vi "BonOMM-SAOMM.vi"() -> ()   [LabVIEW 2019] (continued)
                        n3249 = control-ref of="TERMINAL"() -> (w7474:refnum<vi>)
                        n3250 = control-ref of="Indicateur d'état"() -> (w7473:refnum<vi>)
                        n3251 = Concatenate Strings("Chargement de la librairie \"", w7468, "\"") -> (w7471:string)
                        n3252 = call "TERMINAL.vi"("Indicateur Refnum"=w7473, "Terminal Refnum"=w7474, "Indicateur d'état"=w7471) -> ()
                      }
                    }
                  }
                }
              }
              event "modify-librairy": Value Change {
                n3253 = event-data() -> ()  [unwired: 1 in, 6 out]
                n3254 = case shown="Vrai" "modify-librairy" {
                  frame False {
                  }
                  frame True {
                    n3255 = local read "loaded_lib"() -> (w7495:path)
                    n3256 = call "Liste-maker.vi"("Path"=w7495) -> ("Save Path"=w7488:path)
                    n3257 = local read "LST"() -> (w7496:dbl)
                    n3258 = call "Read_obs_files.vi"("Path"=w7488) -> ("path used"=w7487:path, "Output Table"=w7498:string[][])
                    n3259 = for {
                      tunnel: w7498 -> [w7504] mode=indexing
                      tunnel: w7496 -> [w7505]
                      tunnel: [w7501] -> w7497 mode=indexing
                      n3260 = Index Array(array=w7504, index #1=2 ("index"), index #2=3 ("index")) -> (element #1=w7507:string, element #2=w7506:string)
                      n3261 = call "Airmass.vi"("temps sidéral"=w7505, "DEC"=w7506, "RA"=w7507) -> ("airmass"=w7502:dbl)
                      n3262 = Number To Fractional String(number=w7502, precision (6)=i16 2) -> (F-format string=w7503:string)  [unwired: 2 in]
                      n3263 = Insert Into Array(array=w7504, index=5, new element=w7503) -> (w7501:string[])
                    }
                    n3264 = local write "loaded_lib"(w7487) -> ()
                    n3265 = Path To String(path=w7487) -> (string=w7489:string)
                    n3266 = local write "Librairie des objets"(w7497) -> ()
                    n3267 = control-ref of="TERMINAL"() -> (w7491:refnum<vi>)
                    n3268 = control-ref of="Indicateur d'état"() -> (w7490:refnum<vi>)
                    n3269 = Concatenate Strings("Modification de la librairie \"", w7489, "\"") -> (w7494:string)
                    n3270 = call "TERMINAL.vi"("Indicateur Refnum"=w7490, "Terminal Refnum"=w7491, "Indicateur d'état"=w7494) -> ()
                  }
                }
              }
              event "Rechercher...": Mouse Down {
                n3271 = event-data() -> ()  [unwired: 1 in, 8 out]
                n3272 = while {
                  stop <- w7516 continue-if-true
                  n3273 = local read "Librairie complète"() -> (w7511:string[][])
                  n3274 = local read "Rechercher..."() -> (w7514:string)
                  n3275 = call "Update_library.vi"("Librairie des objets"=w7511, "String to Search"=w7514) -> ("lib_out"=w7513:string[][])
                  n3276 = local read "Classé par ..."() -> (w7515:i32)
                  n3277 = Wait (ms)(milliseconds to wait=u32 25) -> ()  [unwired: 1 out]
                  n3278 = call "Sort_table.vi"("Column"=w7515, "Table-In"=w7513) -> ("Table-Out"=w7512:string[][])
                  n3279 = local write "Librairie des objets"(w7512) -> ()
                  n3280 = property on="Rechercher..." class="Ch"() -> ("Key Focus"=w7516:bool)  [unwired: 2 in, 2 out]
                }
              }
              event "Classé par ...": Value Change {
                n3281 = event-data() -> ()  [unwired: 1 in, 6 out]
                n3282 = local read "Librairie des objets"() -> (w7519:string[][])
                n3283 = local read "Classé par ..."() -> (w7517:i32)
                n3284 = call "Sort_table.vi"("Column"=w7517, "Table-In"=w7519) -> ("Table-Out"=w7518:string[][])
                n3285 = local write "Librairie des objets"(w7518) -> ()
              }
              event "centrer_curseur_table": Value Change {
                n3286 = event-data() -> ()  [unwired: 1 in, 6 out]
                n3287 = case shown="Vrai" "centrer_curseur_table" {
                  frame False {
                  }
                  frame True {
                    n3288 = property on="TableXYPos" class="GraphXY (strict)"("Active Cursor"=u32 1 ("Cursor.Cursor Index")) -> (error out=w7524:errorcluster, "Cursor.Cursor Position"=w7522:T45)  [unwired: 2 in, 1 out]
                    n3289 = local write "centrer_curseur_table"(FALSE) -> ()
                    n3290 = property on="TableXYPos" class="GraphXY (strict)"(error in=w7524, "Active Cursor"=u32 0 ("Cursor.Cursor Index"), "Cursor.Cursor Position"=w7522) -> ()  [unwired: 1 in, 2 out]
                  }
                }
              }
              event "centrer_curseur": Value Change {
                n3291 = event-data() -> ()  [unwired: 1 in, 6 out]
                n3292 = local write "centrer_curseur"(FALSE ("centrer_curseur")) -> ()
                n3293 = flat-sequence {
                  frame #0 {
                    n3294 = local write "CursorLock"(TRUE ("CursorLock")) -> ()
                  }
                  frame #1 {
                    n3295 = property on="TableXYPos" class="GraphXY (strict)"() -> ("XScale.Maximum"=w7535:dbl, "XScale.Minimum"=w7534:dbl)  [unwired: 2 in, 2 out]
                    n3296 = property on="TableXYPos" class="GraphXY (strict)"() -> ("YScale.Maximum"=w7531:dbl, "YScale.Minimum"=w7530:dbl)  [unwired: 2 in, 2 out]
                    n3297 = Add(x=w7535, y=w7534) -> (x+y=w7536:dbl)
                    n3298 = Add(x=w7531, y=w7530) -> (x+y=w7532:dbl)
                    n3299 = expression code="x/2"(w7536) -> (w7533:dbl)
                    n3300 = expression code="x/2"(w7532) -> (w7529:dbl)
                    n3301 = property on="TableXYPos" class="GraphXY (strict)"("Active Cursor"=u32 0, "Cursor.Cursor X"=w7533, "Cursor.Cursor Y"=w7529) -> ()  [unwired: 2 in, 2 out]
                  }
                  frame #2 {
                    n3302 = local write "CursorLock"(FALSE ("CursorLock")) -> ()
                  }
                }
              }
              event "SaveExcpt": Value Change {
                n3303 = event-data() -> ()  [unwired: 1 in, 6 out]
                n3304 = case shown="Faux" "SaveExcpt" {
                  frame False {
                  }
                  frame True {
                    n3305 = global read "Globals.vi" "BonOMM VI Refnum"() -> (w7545:refnum<vi>)
                    n3306 = invoke class="VI" method="ValCmde.ToutObt (obs)"(reference=w7545, "controls"=FALSE) -> (reference out=w7544:refnum<vi>, error out=w7543:errorcluster, "Get All Control Values"=w7540:T46)  [unwired: 2 in, 1 out]
                    n3307 = invoke class="VI" method="ValCmde.ToutObt (obs)"(reference=w7544, error in=w7543, "controls"=TRUE) -> ("Get All Control Values"=w7539:T46)  [unwired: 1 in, 3 out]
                    n3308 = call "Save_Params.vi"("Indicators"=w7540, "Controls"=w7539) -> ()  [unwired: 1 in, 1 out]
                  }
                }
              }
              event "Offset RA", "Offset DEC": Value Change; "OffRA_dir", "OffDEC_dir": Mouse Down {
                n3309 = event-data() -> ("CtlRef"=w7553:refnum<vi>)  [unwired: 1 in, 3 out]
                n3310 = property class="Cmde"(reference=w7553) -> ("Label.Text"=w7552:string)  [unwired: 1 in, 2 out]
                n3311 = local read "Offset DEC"() -> (w7550:dbl)
                n3312 = local read "Offset RA"() -> (w7551:dbl)
                n3313 = case shown="\"OffDEC_dir\"" w7552 {
                  tunnel: w7551 -> [w7555 w7556 w7560]
                  tunnel: w7550 -> [w7554 w7558 w7561]
                  tunnel: [w7555 w7556 w7559] -> w7547
                  tunnel: [w7554 w7557 w7561] -> w7546
                  frame "Offset A.D.", "Offset Déc.", Default {
                  }
                  frame "OffDEC_dir" {
                    n3314 = Negate(x=w7558) -> (-x=w7557:dbl)
                    n3315 = local write "Offset DEC"(w7557) -> ()
                    n3316 = local write "Offset RA"(w7556) -> ()
                  }
                  frame "OffRA_dir" {
                    n3317 = Negate(x=w7560) -> (-x=w7559:dbl)
                    n3318 = local write "Offset DEC"(w7561) -> ()
                    n3319 = local write "Offset RA"(w7559) -> ()
                  }
                }
                n3320 = call "Set_Offset_dir.vi"("DEC"=w7546, "RA"=w7547) -> ("DEC_dir"=→"OffDEC_dir":string, "RA_dir"=→"OffRA_dir":string)
              }
              event "Offset RA", "Offset DEC": Mouse Down {
                n3321 = event-data() -> ()  [unwired: 1 in, 8 out]
              }
              event "copy_calib", "copy_ref", "copy_centre": Value Change {
                n3322 = event-data() -> ("CtlRef"=w7570:refnum<vi>)  [unwired: 1 in, 5 out]
                n3323 = property class="Bool"(reference=w7570) -> ("Label.Text"=w7569:string)  [unwired: 1 in, 2 out]
                n3324 = case shown="\"copy_ref\"" w7569 {
                  tunnel: ["<NO REFERENCE>" "de calibration" "de la référence instrumentale" "du centre optique"] -> w7565
                  frame Default {
                  }
                  frame "copy_calib" {
                  }
                  frame "copy_ref" {
                  }
                  frame "copy_centre" {
                  }
                }
                n3325 = Concatenate Strings("Êtes vous certain de vouloir modifier la position ", w7565, " ?") -> (w7564:string)
                n3326 = Two Button Dialog(message=w7564, 1:"NON" ("T button name (\"OK\")"), 2:"OUI" ("T button name (\"OK\")")) -> (T button?=w7568:bool)
                n3327 = case shown="Vrai" w7568 {
                  tunnel: w7569 -> [_ w7571]
                  frame False {
                  }
                  frame True {
                    n3328 = local read "Position X"() -> (w7574:dbl)
                    n3329 = local read "Position Y"() -> (w7573:dbl)
                    n3330 = local read "Position Z"() -> (w7572:dbl)
                    n3331 = case shown="\"copy_centre\"" w7571 {
                      tunnel: w7574 -> [_ w7576 w7578 w7580]
                      tunnel: w7573 -> [_ w7575 w7577 w7579]
                      tunnel: w7572 -> [_ _ _ _]
                      frame Default {
                      }
                      frame "copy_calib" {
                        n3332 = local write "Calibration X"(w7576) -> ()
                        n3333 = local write "Calibration Y"(w7575) -> ()
                      }
                      frame "copy_ref" {
                        n3334 = local write "Reference X"(w7578) -> ()
                        n3335 = local write "Reference Y"(w7577) -> ()
                      }
                      frame "copy_centre" {
                        n3336 = local write "CentreTel X"(w7580) -> ()
                        n3337 = local write "CentreTel Y"(w7579) -> ()
                      }
                    }
                  }
                }
              }
              event "Cen-Snd-RA", "Cen-Snd-DEC", "Cen-Cib-RA", "Cen-Cib-DEC": Value Change {
                n3338 = event-data() -> ()  [unwired: 1 in, 6 out]
                n3339 = disable-structure shown="Disabled" {
                  frame Disabled {
                    n3340 = local read "Cen-Snd-DEC"() -> ()  [unwired: 1 out]
                    n3341 = local read "Cen-Snd-RA"() -> ()  [unwired: 1 out]
                  }
                  frame Enabled {
                  }
                }
                n3342 = call "format_string2arcmin.vi"("Arcmin-Str"="Cen-Cib-DEC") -> ("Arcmin"=w7588:dbl)  [unwired: 14 in]
                n3343 = call "format_string2arcmin.vi"("Arcmin-Str"="Cen-Cib-RA") -> ("Arcmin"=w7589:dbl)  [unwired: 14 in]
                n3344 = property on="TableXYPos" class="GraphXY (strict)"("Active Cursor"=u32 0, "Cursor.Cursor X"=w7589, "Cursor.Cursor Y"=w7588) -> ()  [unwired: 2 in, 2 out]
              }
              event "best_target": Value Change {
                # "Remettre les conditions sur BestTargetLed"
                n3345 = event-data() -> ()  [unwired: 1 in, 6 out]
                n3346 = stacked-sequence {
                  frame #0 {
                    n3347 = local write "best_target"(FALSE ("best_target")) -> ()
                    n3348 = property on="best_target" class="Bool (strict)"("DisabledEnum"=T17."Disabled" ("Disabled")) -> ()  [unwired: 2 in, 2 out]
                  }
                  frame #1 {
                    # "Vérifie si le data est à date ..."
                    n3349 = local read "BestTargetLed"() -> (w7592:bool)
                    n3350 = case shown="Faux" w7592 {
                      frame False {
                        n3351 = local read "DEC-Champ"() -> (w7594:dbl)
                        n3352 = local read "RA-Champ"() -> (w7595:dbl)
                        n3353 = local write "BestTargetLed"(FALSE ("BestTargetLed")) -> ()
                        n3354 = flat-sequence {
                          tunnel: [w7604] -> w7596
                          tunnel: w7595 -> [w7601]
                          tunnel: w7594 -> [w7600]
                          tunnel: w7596 -> [w7622]
                          frame #0 {
                            # "R1mag limite USNO"
                            n3355 = local read "Représentation"() -> (w7599:dbl)
                            n3356 = local read "path_data"() -> (w7606:path)
                            n3357 = local read "wgetexec"() -> (w7605:path)
                            n3358 = Add(x=w7599, y=10.0) -> (x+y=w7597:dbl)
                            n3359 = while {
                              stop <- w7610 stop-if-true
                              n3360 = local read "BestTargetLed"() -> (w7612:bool)
                              n3361 = Wait (ms)(milliseconds to wait=u32 333) -> ()  [unwired: 1 out]
                              n3362 = Not(x=w7612) -> (.not. x?=w7611:bool)
                              n3363 = local write "BestTargetLed"(w7611) -> ()
                              n3364 = local read "USNO_ready"() -> (w7610:bool)
                            }
                            n3365 = call "QueryUSNO.vi"("wget"=w7605, "Data dir Path"=w7606, "mag_limit"=12.0, "radius"=w7597, "DEC"=w7600, "RA"=w7601) -> ("Data OUT"=w7607:string[][], "No Error"=w7602:bool)  [unwired: 3 in, 1 out]
                            n3366 = case shown="Vrai" w7602 {
                              tunnel: w7607 -> [_ w7621]
                              tunnel: w7602 -> [w7614 w7619]
                              tunnel: [w7614 w7619] -> w7604
                              tunnel: [TRUE TRUE] -> w7603
                              tunnel: w7601 -> [_ w7616]
                              tunnel: w7600 -> [_ w7615]
                              frame False {
                              }
                              frame True {
                                # "6 = R1mag"
                                n3367 = call "Sort_USNO_data.vi"("Column Used"=6, "Data IN"=w7621) -> ("Data OUT"=w7617:string[][])  [unwired: 8 in, 1 out]
                                n3368 = local write "USNO_data"(w7617) -> ()
                                "RA-USNO" <- w7616
                                "DEC-USNO" <- w7615
                              }
                            }
                            n3369 = local write "USNO_ready"(w7603) -> ()
                          }
                          frame #1 {
                            n3370 = local write "USNO_ready"(w7622) -> ()
                            "BestTargetLed" <- w7622
                          }
                        }
                      }
                      frame True {
                      }
                    }
                  }
                  frame #2 {
                    n3371 = local read "BestTargetLed"() -> (w7623:bool)
                    n3372 = case shown="Vrai" w7623 {
                      frame False {
                      }
                      frame True {
                        w7624 = u16 1 items=["Region d'intérêt", "Prévisualisation", "Idle"] ("ImageUsage")
                        # "Proper motion limit (mas/yr)"
                        # "Pickup mirror footprint (arcmin)"
                        # "R1mag lower limit"
                        n3373 = local read "FOV"() -> (w7652:dbl)
                        n3374 = local read "TableAstrom"() -> (w7635:T4)
                        n3375 = local read "USNO_data"() -> (w7657:string[][])
                        n3376 = local read "Epoch Tel"() -> (w7654:dbl)
                        n3377 = local read "DEC Tel"() -> (w7655:dbl)
                        n3378 = local read "RA Tel"() -> (w7656:dbl)
                        n3379 = call "Choose_best_target(multi).vi"("R1mag lower limit"=6.0, "FOV"=w7652, "Footprint"=1.0, "PM limit"=25.0 ("Footprint"), "EPOCH TEL"=w7654, "DEC TEL"=w7655, "Table Astrometry"=w7635, "RA TEL"=w7656, "USNO_data"=w7657) -> ("Best Target"=w7634:string[][], "target RA (deg)"=w7643:dbl, "target DEC (deg)"=w7642:dbl)  [unwired: 3 in, 5 out]
                        "Target Data" <- w7634
                        n3380 = local read "FirstBest"() -> (w7641:bool)
                        n3381 = case shown="Faux" w7641 {
                          selector: w7641 -> [_ w7675]
                          tunnel: w7643 -> [_ w7677]
                          tunnel: [w7661 w7677] -> w7631
                          tunnel: w7642 -> [_ w7676]
                          tunnel: [w7660 w7676] -> w7630
                          tunnel: w7634 -> [w7672 _]
                          frame False {
                            n3382 = Increment(x="BestCount") -> (x+1=w7668:i32)
                            n3383 = Index Array(array=w7672, index (row)="BestCount") -> (element=w7669:string[])  [unwired: 1 in]
                            n3384 = Quotient & Remainder(x=w7668, y=3) -> (x-y*floor(x/y)=w7671:i32)  [unwired: 1 out]
                            n3385 = Index Array(array=w7669) -> (element #1=w7667:string, element #2=w7666:string, element #3=w7665:string)  [unwired: 3 in]
                            n3386 = local read "Epoch Tel"() -> (w7658:dbl)
                            n3387 = Fract/Exp String To Number(string=w7667) -> (number=w7664:dbl)  [unwired: 3 in, 1 out]
                            n3388 = Fract/Exp String To Number(string=w7666) -> (number=w7663:dbl)  [unwired: 3 in, 1 out]
                            n3389 = Fract/Exp String To Number(string=w7665) -> (number=w7662:dbl)  [unwired: 3 in, 1 out]
                            n3390 = local write "BestCount"(w7671) -> ()
                            n3391 = call "precess.vi"("Eq2"=w7658, "Eq1"=w7662, "DEC 1"=w7663, "RA 1"=w7664) -> ("DEC 2"=w7660:dbl, "RA 2"=w7661:dbl)
                          }
                          frame True {
                            n3392 = Not(x=w7675) -> (.not. x?=→"FirstBest":bool)
                            n3393 = local write "BestCount"(1 ("BestCount")) -> ()
                          }
                        }
                        n3394 = local read "ImageDSSLed"() -> (w7644:bool)
                        n3395 = local read "Epoch Tel"() -> (w7628:dbl)
                        n3396 = call "precess.vi"("Eq2"=2000.0, "Eq1"=w7628, "DEC 1"=w7630, "RA 1"=w7631) -> ("DEC 2"=w7626:dbl, "RA 2"=w7627:dbl)
                        n3397 = call "deg2ad.vi"("DEC (°)"=w7630, "RA (°)"=w7631) -> ("DEC (°)"=→"RA-USNO-sec 3":dbl, "RA (sec)"=→"RA-USNO-sec 2":dbl)
                        n3398 = case shown="Faux" w7644 {
                          tunnel: w7627 -> [w7682 w7701]
                          tunnel: w7626 -> [w7681 w7700]
                          tunnel: [w7679 w7699] -> w7646
                          frame False {
                            w7683 = 2.0 ("Size")
                            n3399 = local read "wgetexec"() -> (w7685:path)
                            n3400 = local read "path_dss"() -> (w7684:path)
                            n3401 = call "Query_Vizier.vi"("Folder"=w7684, "wget"=w7685, "Width"=w7683, "Height"=w7683, "DEC"=w7681, "RA"=w7682) -> ("error?"=w7678:bool, "Path2Image"=w7680:path)  [unwired: 4 in]
                            n3402 = case shown="Faux" w7678 {
                              tunnel: w7680 -> [w7690 _]
                              tunnel: [w7689 w7697] -> w7679
                              frame False {
                                n3403 = call "gfitsio-open-create-replace-file.vi"("file path (dialog if empty)"=w7690) -> ("error out"=w7695:errorcluster, "gfits refnum"=w7694:T47)  [unwired: 8 in, 1 out]
                                n3404 = call "gfitsio-read-header.vi"("error in (no error)"=w7695, "gfits refnum"=w7694) -> ("error out"=w7692:errorcluster, "dup gfits refnum"=w7693:T47)  [unwired: 7 in, 1 out]
                                n3405 = call-poly "gfitsio-read-image-subset.vi"("lpixel (-1,-1: rest)"=cluster{"X":i32, "Y":i32} {"X"=-1, "Y"=-1}, "fpixel (1,1)"=cluster{"X":i32, "Y":i32} {"X"=1, "Y"=1}, "error in (no error)"=w7692, "gfits refnum"=w7693) -> ("error out"=w7688:errorcluster, "data"=w7689:sgl[][], "dup gfits refnum"=w7687:T47)  [unwired: 4 in, 1 out]
                                n3406 = call "gfitsio-close-file.vi"("error in (no error)"=w7688, "gfits refnum"=w7687) -> ("error out"=→"fits Error":errorcluster)  [unwired: 8 in, 1 out]
                              }
                              frame True {
                                w7698 = sgl 0.0 ("element")
                                n3407 = Initialize Array(w7698, w7698, w7698) -> (w7697:sgl[][])
                              }
                            }
                          }
                          frame True {
                            n3408 = local read "ImgAstrom"() -> (w7709:T4)
                            n3409 = call "ad2xy.vi"("DEC"=w7700, "RA"=w7701, "Astrometry"=w7709) -> ("Y"=w7706:dbl, "X"=w7707:dbl)  [unwired: 6 in, 1 out]
                            n3410 = To Long Integer(number=w7707) -> (32bit integer=w7705:i32)
                            n3411 = To Long Integer(number=w7706) -> (32bit integer=w7704:i32)
                            n3412 = local read "ImgData"() -> (w7708:sgl[][])
                            n3413 = call "subimage.vi"("Ysz/2"=100, "Xsz/2"=100, "Yc"=w7704, "Xc"=w7705, "ImgData"=w7708) -> ("SubImg"=w7699:sgl[][])  [unwired: 6 in]
                          }
                        }
                        n3414 = local read "FieldAstrom"() -> (w7648:T4)
                        n3415 = local write "SubIMG4DSS?"(TRUE ("SubIMG4DSS?")) -> ()
                        n3416 = call "ad2xy.vi"("DEC"=w7630, "RA"=w7631, "Astrometry"=w7648) -> ("Y"=w7636:dbl, "X"=w7637:dbl)  [unwired: 6 in, 1 out]
                        n3417 = property on="TableXYPos" class="GraphXY (strict)"("Active Cursor"=u32 0, "Cursor.Cursor Position:Cursor X"=w7637, "Cursor.Cursor Position:Cursor Y"=w7636) -> ()  [unwired: 2 in, 2 out]
                        n3418 = call "format_arcmin2arcsecstr.vi"("RA arcmin"=w7637, "DEC Arcmin"=w7636) -> ("Formatted RA"=w7640:string, "Formatted Dist"=w7638:string, "Formatted DEC"=w7639:string)  [unwired: 11 in]
                        n3419 = Array Max & Min(array=w7646) -> (max value=w7647:sgl)  [unwired: 3 out]
                        n3420 = call "Draw_crosshair.vi"("Image IN"=w7646, "White Value"=w7647) -> ("Image OUT"=w7645:sgl[][])  [unwired: 13 in]
                        n3421 = local write "Cen-Cib-TOT"(w7638) -> ()
                        n3422 = local write "Cen-Cib-RA"(w7640) -> ()
                        n3423 = local write "Cen-Cib-DEC"(w7639) -> ()
                        n3424 = local write "ImageUsage"(w7624) -> ()
                        n3425 = local write "subimg"(w7645) -> ()
                      }
                    }
                  }
                  frame #3 {
                    n3426 = property on="best_target" class="Bool (strict)"("DisabledEnum"=T17."Enabled" ("Disabled")) -> ()  [unwired: 2 in, 2 out]
                  }
                }
              }
              event "GetDSS", "DS9": Value Change {
                # "Trace l'image DSS par dessus le champ des tables de guidage"
                n3427 = event-data() -> ("CtlRef"=w7715:refnum<vi>)  [unwired: 1 in, 4 out]
                n3428 = flat-sequence {
                  tunnel: w7715 -> [w7721]
                  tunnel: [w7720] -> w7714
                  tunnel: [w7753] -> w7717
                  tunnel: w7714 -> [w7747]
                  tunnel: [w7741] -> w7713
                  tunnel: [w7740] -> w7712
                  tunnel: [w7739] -> w7711
                  tunnel: w7717 -> [w7810]
                  tunnel: path "C:/BonOMM/BonOMM-2012/Apps/SAOImage-DS9/ds9.exe" ("DS9path") -> [w7809]
                  tunnel: w7713 -> [w7805]
                  tunnel: w7712 -> [w7807]
                  tunnel: w7711 -> [w7806]
                  frame #0 {
                    w7719 = T17."Disabled" ("Disabled")
                    w7718 = FALSE ("DSS_ready")
                    n3429 = property class="Bool (strict)"(reference=w7721) -> ("Label.Text"=w7720:string)  [unwired: 1 in, 2 out]
                    n3430 = local write "ImageDSSLed"(w7718) -> ()
                    n3431 = local write "DS9-Led"(w7718) -> ()
                    n3432 = local write "DSS_ready"(w7718) -> ()
                    n3433 = local write "DS9_ready"(w7718) -> ()
                    n3434 = local write "GetDSS"(w7718) -> ()
                    n3435 = property on="DS9" class="Bool (strict)"("DisabledEnum"=w7719) -> ()  [unwired: 2 in, 2 out]
                    n3436 = property on="GetDSS" class="Bool (strict)"("DisabledEnum"=w7719) -> ()  [unwired: 2 in, 2 out]
                    n3437 = local write "DS9"(w7718) -> ()
                  }
                  frame #1 {
                    w7772 = u16 0 items=["Square", "Circle"] ("Ring")
                    # "Invert X"
                    # "Époque DSS et USNO"
                    n3438 = local read "Reference Y"() -> (w7774:dbl)
                    n3439 = local read "Reference X"() -> (w7773:dbl)
                    n3440 = local read "CentreTel X"() -> (w7737:dbl)
                    n3441 = local read "CentreTel Y"() -> (w7736:dbl)
                    n3442 = local read "RotationEffective"() -> (w7733:dbl)
                    n3443 = local read "arcsec/pulse"() -> (w7770:dbl)
                    n3444 = local read "Représentation"() -> (w7746:dbl)
                    n3445 = To Double Precision Float(number=w7773) -> (double precision float=w7765:dbl)
                    n3446 = To Double Precision Float(number=w7774) -> (double precision float=w7764:dbl)
                    n3447 = Equal?(x=w7747, y="DS9") -> (x = y?=w7741:bool)
                    n3448 = Select(t=60.0, s=w7741, f=w7746) -> (s? t:f=w7745:dbl)
                    n3449 = local read "DEC Tel"() -> (w7767:dbl)
                    n3450 = local read "RA Tel"() -> (w7766:dbl)
                    n3451 = while {
                      tunnel: w7747 -> [w7775]
                      stop <- w7777 stop-if-true
                      n3452 = case shown="\"DS9\"" w7775 {
                        tunnel: [TRUE ("DSS_ready") w7781 "DS9_ready"] -> w7777
                        frame "False", Default {
                        }
                        frame "GetDSS" {
                          n3453 = local read "ImageDSSLed"() -> (w7779:bool)
                          n3454 = local read "DSS_ready"() -> (w7781:bool)
                          n3455 = Not(x=w7779) -> (.not. x?=→"ImageDSSLed":bool)
                        }
                        frame "DS9" {
                          n3456 = local read "DS9-Led"() -> (w7783:bool)
                          n3457 = Not(x=w7783) -> (.not. x?=→"DS9-Led":bool)
                        }
                      }
                      n3458 = Wait (ms)(milliseconds to wait=u32 333) -> ()  [unwired: 1 out]
                    }
                    n3459 = call "Set_field_astrometry.vi"("Cen x (pas)"=w7737, "effective rotation (°)"=w7733, "scale (\"/pas)"=w7770, "NaxisMax"=500000, "Cen y (pas)"=w7736, "Use Center?"=FALSE ("Ues Constant Size ?"), "Ref x (pas)"=w7765, "Ref y (pas)"=w7764, "RA (HH:MM:SS.S)"=w7766, "DEC(DD:MM:SS)"=w7767, "Inversion Cluster"=T20 {"Invert Angle"=FALSE, "Invert X"=TRUE, "Invert Y"=FALSE}) -> ("Field Astrometry"=w7759:T4, "Table Astrometry"=w7760:T4)  [unwired: 3 in]
                    n3460 = local read "MirVig"() -> (w7730:dbl)
                    n3461 = property on="TableXYPos" class="GraphXY (strict)"("Active Cursor"=u32 1) -> ("Cursor.Cursor X"=w7728:dbl, "Cursor.Cursor Y"=w7729:dbl)  [unwired: 2 in, 2 out]
                    n3462 = local read "BrasPesto"() -> (w7722:bool)
                    n3463 = local read "LimXPesto"() -> (w7723:dbl)
                    n3464 = local read "MirFOV"() -> (w7725:dbl)
                    n3465 = local read "Miroir"() -> (w7727:dbl)
                    n3466 = local read "FOV"() -> (w7771:dbl)
                    n3467 = local write "TableAstrom"(w7760) -> ()
                    n3468 = local read "NaxisMax"() -> (w7738:dbl)
                    n3469 = Bundle("Miroir"=w7727, "Cursor.Cursor X"=w7728, "Cursor.Cursor Y"=w7729, "MirVig"=w7730, "MirFOV"=w7725, "LimXPesto"=w7723, "BrasPesto"=w7722) -> (w7726:T48)  [unwired: 1 in]
                    n3470 = local read "RotationEffective"() -> (w7724:dbl)
                    n3471 = local read "Epoch Tel"() -> (w7757:dbl)
                    n3472 = call "draw_field.vi"("Field_Astrometry"=w7759, "FOV"=w7771, "NaxisMax"=w7738, "Ring"=w7772, "Table_Astrometry"=w7760, "Rotation effective"=w7724, "Ues Constant Size ?"=TRUE, "margin/size"=w7745, "MirrorAvatar"=w7726) -> ("X Scale.Range"=w7752:T26, "ImgDEC"=w7732:dbl, "ImgRA"=w7756:dbl, "Y Scale.Range"=w7751:T26)  [unwired: 2 in, 1 out]
                    n3473 = call "precess.vi"("Eq2"=2000.0, "Eq1"=w7757, "DEC 1"=w7732, "RA 1"=w7756) -> ("DEC 2"=w7754:dbl, "RA 2"=w7755:dbl)
                    n3474 = local read "path_dss"() -> (w7762:path)
                    n3475 = Add(x=w7745, y=4.0) -> (x+y=w7750:dbl)
                    n3476 = local read "wgetexec"() -> (w7761:path)
                    n3477 = local write "FieldAstrom"(w7759) -> ()
                    n3478 = call "Query_Vizier.vi"("Folder"=w7762, "wget"=w7761, "Width"=w7750, "Height"=w7750, "DEC"=w7754, "RA"=w7755) -> ("error?"=w7742:bool, "Path2Image"=w7763:path)  [unwired: 4 in]
                    n3479 = local write "Img DEC"(w7754) -> ()
                    n3480 = local write "Img RA"(w7755) -> ()
                    n3481 = Or(x=w7742, y=w7741) -> (x .or. y?=w7743:bool)
                    n3482 = case shown="Faux" w7743 {
                      tunnel: w7755 -> [w7797 _]
                      tunnel: w7754 -> [w7796 _]
                      tunnel: w7763 -> [w7788 w7803]
                      tunnel: w7759 -> [w7794 _]
                      tunnel: [TRUE TRUE] -> w7740
                      tunnel: [w7788 w7803] -> w7753
                      tunnel: w7752 -> [w7787 _]
                      tunnel: w7751 -> [w7786 _]
                      tunnel: [w7785 FALSE] -> w7739
                      frame False {
                        # "ImgData et ImgAstrom\nsont lié à plus grand que le\nchamp affiché."
                        n3483 = property on="TableXYPos" class="GraphXY (strict)"() -> ("Height"=w7801:u32, "Width"=w7800:u32)  [unwired: 2 in, 2 out]
                        n3484 = To Long Integer(number=w7801) -> (32bit integer=w7799:i32)
                        n3485 = To Long Integer(number=w7800) -> (32bit integer=w7798:i32)
                        n3486 = call "Draw_graph_background.vi"("Y Scale.Range"=w7786, "ImgRA"=w7797, "X Scale.Range"=w7787, "ImgDEC"=w7796, "Field Astrometry"=w7794, "New Width"=w7798, "New Height"=w7799, "path"=w7788) -> ("ImgData"=w7789:sgl[][], "Astrometry"=w7793:T4, "error out"=w7791:errorcluster, "Images"=w7795:picture)
                        "DSS Error" <- w7791
                        n3487 = Unbundle By Name(w7791) -> ("status"=w7790:bool)
                        n3488 = property on="TableXYPos" class="GraphXY (strict)"("PlotImages.Back"=w7795) -> ()  [unwired: 2 in, 2 out]
                        n3489 = local write "ImgAstrom"(w7793) -> ()
                        n3490 = local write "ImgData"(w7789) -> ()
                        n3491 = Not(x=w7790) -> (.not. x?=w7785:bool)
                      }
                      frame True {
                      }
                    }
                    n3492 = local write "DSS_ready"(w7740) -> ()
                    n3493 = local write "DS9_ready"(w7740) -> ()
                  }
                  frame #2 {
                    w7808 = T17."Enabled" ("Disabled")
                    n3494 = property on="GetDSS" class="Bool (strict)"("DisabledEnum"=w7808) -> ()  [unwired: 2 in, 2 out]
                    n3495 = case shown="Vrai" w7805 {
                      tunnel: w7810 -> [_ w7814]
                      tunnel: w7809 -> [_ w7813]
                      tunnel: w7807 -> [_ w7812]
                      tunnel: w7806 -> [w7811 _]
                      frame False {
                        n3496 = local write "ImageDSSLed"(w7811) -> ()
                      }
                      frame True {
                        n3497 = local write "DS9-Led"(w7812) -> ()
                        n3498 = call "fits2ds9.vi"("DS9path"=w7813, "FitsFile"=w7814) -> ()  [unwired: 10 in]
                      }
                    }
                    n3499 = property on="DS9" class="Bool (strict)"("DisabledEnum"=w7808) -> ()  [unwired: 2 in, 2 out]
                  }
                }
              }
              event "BoutonTest": Value Change {
                n3500 = event-data() -> ()  [unwired: 1 in, 6 out]
                n3501 = flat-sequence {
                  frame #0 {
                    n3502 = local write "QueryingHexapod"(TRUE ("QueryingHexapod")) -> ()
                    n3503 = property on="HexapodRefresh" class="Bool (strict)"("Val(Sgnl)"=TRUE ("Valeur (Signalisation)")) -> ()  [unwired: 2 in, 2 out]
                  }
                  frame #1 {
                    n3504 = while {
                      i -> [w7821]
                      stop <- w7818 stop-if-true
                      n3505 = local read "QueryingHexapod"() -> (w7822:bool)
                      n3506 = Not(x=w7822) -> (.not. x?=w7820:bool)
                      n3507 = call "Max-iteration.vi"("i max"=50, "i act"=w7821, "Valeur entrante"=w7820) -> ("break ?"=w7818:bool)
                      n3508 = Wait (ms)(milliseconds to wait=u32 100 ("attente (ms)")) -> ()  [unwired: 1 out]
                    }
                    n3509 = local write "GE_Hex_X"(0.01 ("GE_Hex_X")) -> ()
                  }
                  frame #2 {
                    n3510 = local read "GE_Hex_Y"() -> (w7828:dbl)
                    n3511 = local read "GE_Hex_U"() -> (w7826:dbl)
                    n3512 = local read "GE_Hex_X"() -> (w7829:dbl)
                    n3513 = local read "GE_Hex_Z"() -> (w7827:dbl)
                    n3514 = local read "GE_Hex_V"() -> (w7825:dbl)
                    n3515 = local read "Hexapod VRN"() -> (w7833:refnum<visa-resource-name>)
                    n3516 = control-ref of="HexX"() -> (w7840:refnum<vi>)
                    n3517 = control-ref of="HexY"() -> (w7839:refnum<vi>)
                    n3518 = control-ref of="HexU"() -> (w7837:refnum<vi>)
                    n3519 = control-ref of="HexV"() -> (w7836:refnum<vi>)
                    n3520 = control-ref of="HexZ"() -> (w7838:refnum<vi>)
                    n3521 = control-ref of="Hexapod-ACK"() -> (w7831:refnum<vi>)
                    n3522 = control-ref of="HexaCons actif"() -> (w7832:refnum<vi>)
                    n3523 = local read "MessageType"() -> (w7834:cluster{string[], u32[]})
                    n3524 = Bundle("GE_Hex_X"=w7829, "GE_Hex_Y"=w7828, "GE_Hex_Z"=w7827, "GE_Hex_U"=w7826, "GE_Hex_V"=w7825) -> (w7824:T49)  [unwired: 1 in]
                    n3525 = Bundle("HexX"=w7840, "HexY"=w7839, "HexZ"=w7838, "HexU"=w7837, "HexV"=w7836) -> (w7835:T29)  [unwired: 1 in]
                    n3526 = call "TEST-SAOMM-Externaloffset.vi"("Hexapod VRN"=w7833, "Active Refnum"=w7832, "PrAMS-ACK"=w7831, "output cluster"=w7835, "offset_cluster"=w7824, "MessageType"=w7834) -> ("Error"=w7830:bool)  [unwired: 9 in]
                    n3527 = case shown="Vrai" w7830 {
                      frame False {
                      }
                      frame True {
                        n3528 = One Button Dialog(message="Erreur lors de l'envoi des valeurs offset 2") -> ()  [unwired: 1 in, 1 out]
                      }
                    }
                  }
                }
              }
              event "LVDT-Set-ZERO": Value Change {
                n3529 = event-data() -> ()  [unwired: 1 in, 5 out]
                n3530 = local write "LVDT-Set-ZERO"(FALSE ("LVDT-Set-ZERO")) -> ()
                n3531 = flat-sequence {
                  tunnel: [w7846] -> w7842
                  tunnel: w7842 -> [w7847]
                  frame #0 {
                    n3532 = Two Button Dialog(message="Assurez-vous que les moteurs sont éteints depuis au\nmoins 30 secondes et que les plateaux sont bien engagés.", 1:"Annuler" ("F button name (\"Cancel\")")) -> (T button?=w7846:bool)  [unwired: 1 in]
                  }
                  frame #1 {
                    n3533 = case shown="Vrai" w7847 {
                      frame False {
                      }
                      frame True {
                        n3534 = local read "Graph Data"() -> (w7848:dbl[])
                        n3535 = call-poly <vilib>:"Mean.vi"("X"=w7848) -> ("mean"=w7849:dbl)  [unwired: 1 out]
                        n3536 = local write "LVDT-zero"(w7849) -> ()
                      }
                    }
                  }
                }
              }
              event "LVDT-Save-Data": Value Change {
                n3537 = event-data() -> ()  [unwired: 1 in, 5 out]
                n3538 = local write "LVDT-Save-Data"(FALSE ("want seconds? (F)")) -> ()
                n3539 = local read "LVDT-RA-Data"() -> (w7875:dbl[])
                n3540 = local read "Q String"() -> (w7871:string)
                n3541 = Array To Spreadsheet String(delimiter (Tab)="\n", array=w7875, 3:"%5f") -> (spreadsheet string=w7873:string)
                n3542 = Get Date/Time String(date format (0)=enum16{"short", "long", "abbreviated"}."short", want seconds? (F)=TRUE) -> (date string=w7859:string, time string=w7854:string)  [unwired: 1 in]
                n3543 = local read "path_syslogs"() -> (w7869:path)
                n3544 = Search and Replace String(replace all?=TRUE ("replace all? (F)"), input string=w7859, search string="-") -> (result string=w7853:string)  [unwired: 5 in, 3 out]
                n3545 = Search and Replace String(replace all?=TRUE ("replace all? (F)"), input string=w7854, search string=":") -> (result string=w7852:string)  [unwired: 5 in, 3 out]
                n3546 = Concatenate Strings(w7871, "\n\n***\n\n", w7873) -> (w7870:string)
                n3547 = Concatenate Strings(w7853, w7852, ".lvdt" ("name or relative path")) -> (w7862:string)
                n3548 = Build Path(base path=w7869, name or relative path="LVDTs") -> (appended path=w7867:path)
                n3549 = local read "File I/O Error"() -> (w7861:errorcluster)
                n3550 = Build Path(base path=w7867, name or relative path=w7862) -> (appended path=w7866:path)
                n3551 = Write to Text File(file (use dialog)=w7866, text=w7870, error in=w7861) -> (error out=w7860:errorcluster)  [unwired: 1 in, 2 out]
                n3552 = local write "File I/O Error"(w7860) -> ()
              }
              event "SpliterSelector": Value Change {
                n3553 = event-data() -> ("OldVal"=w7878:u16, "NewVal"=w7877:u16)  [unwired: 1 in, 3 out]
                n3554 = Not Equal?(x=w7878, y=w7877) -> (x != y?=w7876:bool)
                n3555 = case shown="Vrai" w7876 {
                  frame False {
                  }
                  frame True {
                    n3556 = flat-sequence {
                      frame #0 {
                        "SplitterMoving" <- TRUE
                      }
                      frame #1 {
                        n3557 = flat-sequence {
                          tunnel: "SpliterSelector" -> [w7885]
                          frame #0 {
                            n3558 = case shown="1" w7885 {
                              tunnel: [w7886 w7891 w7892] -> _
                              frame 2 {
                                w7888 = u16 1 items=["Initialisation", "Mise dans le faisceau", "Retirer du faisceau"] ("Commande")
                                n3559 = local read "Splitter VRN"() -> (w7887:refnum<visa-resource-name>)
                                n3560 = call "MicroSlide-Execute.vi"("VISA resource name"=w7887, "Commande"=w7888) -> ("Error OUT"=w7886:errorcluster)  [unwired: 10 in, 3 out]
                              }
                              frame 0, Default {
                                w7889 = u16 0 items=["Initialisation", "Mise dans le faisceau", "Retirer du faisceau"] ("Commande")
                                n3561 = local read "Splitter VRN"() -> (w7890:refnum<visa-resource-name>)
                                n3562 = call "MicroSlide-Execute.vi"("VISA resource name"=w7890, "Commande"=w7889) -> ("Error OUT"=w7891:errorcluster)  [unwired: 10 in, 3 out]
                              }
                              frame 1 {
                                w7894 = u16 2 items=["Initialisation", "Mise dans le faisceau", "Retirer du faisceau"] ("Commande")
                                n3563 = local read "Splitter VRN"() -> (w7893:refnum<visa-resource-name>)
                                n3564 = call "MicroSlide-Execute.vi"("VISA resource name"=w7893, "Commande"=w7894) -> ("Error OUT"=w7892:errorcluster)  [unwired: 10 in, 3 out]
                              }
                            }
                          }
                          frame #1 {
                            n3565 = local write "SplitterMoving"(FALSE ("SplitterMoving")) -> ()
                          }
                        }
                        n3566 = while {
                          stop <- w7884 continue-if-true
                          n3567 = local read "SpliterIndic"() -> (w7881:bool)
                          n3568 = Wait (ms)(milliseconds to wait=u32 250) -> ()  [unwired: 1 out]
                          n3569 = Not(x=w7881) -> (.not. x?=→"SpliterIndic":bool)
                          n3570 = local read "SplitterMoving"() -> (w7884:bool)
                        }
                      }
                      frame #2 {
                        # "À mettre en gestion d'erreur"
                        n3571 = local write "SpliterIndic"(TRUE ("SpliterIndic")) -> ()
                      }
                    }
                  }
                }
              }
            }
          }
          "Événements Usagés" <- w982
          n3572 = while {
            stop <- w1017 stop-if-true
            # "Boucle d'analyse d'image à haute fréquence ..."
            n3573 = event shown="[0] Timeout" {
              selector: _ -> [_ _]
              dyn-events: _ -> [_ _]
              timeout: 50 -> [_ _]
              event Timeout {
                n3574 = event-data() -> ()  [unwired: 1 in, 2 out]
              }
              event "ProcessImage": Value Change {
                n3575 = event-data() -> ()  [unwired: 1 in, 5 out]
                n3576 = local read "ROIXOffset"() -> (w1025:u16)
                n3577 = local read "ROIYOffset"() -> (w1021:u16)
                n3578 = local write "ProcessImage"(FALSE) -> ()
                n3579 = local read "XCentroid"() -> (w1026:dbl)
                n3580 = local read "YCentroid"() -> (w1022:dbl)
                n3581 = local read "ImageBuffer"() -> (w1038:u16[][])
                n3582 = local read "MaskObjet"() -> (w1039:u8[][])
                n3583 = To Double Precision Float(number=w1025) -> (double precision float=w1024:dbl)
                n3584 = To Double Precision Float(number=w1021) -> (double precision float=w1023:dbl)
                n3585 = Subtract(x=w1026, y=w1024) -> (x-y=w1019:dbl)
                n3586 = Subtract(x=w1022, y=w1023) -> (x-y=w1020:dbl)
                n3587 = local read "PixScale1"() -> (w1041:dbl)
                n3588 = local read "Binning"() -> (w1042:u16)
                n3589 = call "SAOMM-ROI-Stats.vi"("ImageBuffer"=w1038, "ObjectMask"=w1039, "intervals"=32) -> ("ROI Histogram"=→"Histogramme de la ROI":T10, "ImageStat"=w1035:T2)  [unwired: 11 in]
                "ImageStat" <- w1035
                n3590 = To Long Integer(number=w1038) -> (32bit integer=w1028:i32[][])
                n3591 = To Double Precision Float(number=w1042) -> (double precision float=w1040:dbl)
                n3592 = Multiply(x=w1041, y=w1040) -> (x*y=w1030:dbl)
                n3593 = call "PSF-Fitting.vi"("Centoid X"=w1019, "Centroid Y"=w1020, "ROI"=w1028, "''/pix"=w1030) -> ("Credible?"=w1018:bool, "PSF Graph"=w1027:cluster{"PSF X":dbl[], "PSF Y":dbl[]}[], "Seeing"=w1029:dbl)  [unwired: 8 in, 1 out]
                n3594 = case shown="Faux" w1018 {
                  tunnel: w1027 -> [_ w1051]
                  tunnel: w1029 -> [_ w1050]
                  tunnel: [w1045 w1051] -> w1037
                  tunnel: [inf w1050] -> w1036
                  frame False {
                    n3595 = Build Array(0.0) -> (w1047:dbl[])
                    n3596 = Bundle(w1047, w1047) -> (w1046:cluster{dbl[], dbl[]})  [unwired: 1 in]
                    n3597 = Build Array(w1046, w1046) -> (w1045:cluster{dbl[], dbl[]}[])
                  }
                  frame True {
                  }
                }
                "PSF Graph" <- w1037
                "Seeing" <- w1036
                n3598 = Unbundle By Name(w1035) -> ("ObjectMaximumValue"=w1034:dbl)
                n3599 = Greater?(x=w1034, y=50000.0) -> (0:w1032:bool)
                n3600 = property on="Saturé" class="Bool (strict)"("Blinking"=w1032, "Visible"=w1032) -> ()  [unwired: 2 in, 2 out]
              }
            }
            n3601 = local read "Quit"() -> (w1017:bool)
          }
          n3602 = while {
            tunnel: [w2851] -> w970
            stop <- w2851 stop-if-true
            # "Commandes Externes sur le PORT SÉRIE et TCP/IP"
            n3603 = local read "CmdFIFO"() -> (w2852:T14)
            n3604 = Array Size(array=w2852) -> (size(s)=w2854:i32)
            n3605 = Greater Than 0?(x=w2854) -> (x > 0?=w2853:bool)
            n3606 = case shown="Vrai" w2853 {
              tunnel: w2852 -> [_ w2862]
              frame False {
                n3607 = local write "ActiveCmd"(T15 {"CmdAct"="", "CmdArgs"="", "Source"=""} ("ActiveCmd")) -> ()
                "CmdPending" <- FALSE
              }
              frame True {
                w2858 = u32 0 ("Output Code")
                # "Enlève les erreurs ..."
                # "Enlève l'élément du FIFO"
                n3608 = stacked-sequence {
                  tunnel: w2862 -> [_ w2876 _]
                  tunnel: [_ w2871 _] -> w2861
                  tunnel: [_ w2870 _] -> w2860
                  tunnel: [_ w2869 _] -> w2859
                  frame #0 {
                    n3609 = control-ref of="FIFO actif"() -> (w2863:refnum<vi>)
                    n3610 = call "Fifo-Wait4Flag.vi"("Raise Flag ?"=TRUE, "Ctl Refnum IN"=w2863) -> ()  [unwired: 8 in, 2 out]
                  }
                  frame #1 {
                    n3611 = local read "CmdDone"() -> (w2867:T14)
                    n3612 = Delete From Array(array=w2876, length=1, index=0) -> (deleted portion=w2872:T14, array with subset deleted=w2873:T14)
                    n3613 = local write "CmdFIFO"(w2873) -> ()
                    n3614 = Index Array(array=w2872) -> (element=w2868:T15)  [unwired: 1 in]
                    "ActiveCmd" <- w2868
                    n3615 = call "PCE-Archive.vi"("Nouvelle Commande"=w2868, "MaxLength"=3, "CmdDone IN"=w2867) -> ("CmdDone OUT"=w2866:T14)  [unwired: 8 in]
                    n3616 = Unbundle By Name(w2868) -> ("CmdAct"=w2871:string, "CmdArgs"=w2870:string, "Source"=w2869:string)
                    n3617 = local write "CmdDone"(w2866) -> ()
                  }
                  frame #2 {
                    n3618 = local write "FIFO actif"(FALSE) -> ()
                  }
                }
                n3619 = stacked-sequence {
                  tunnel: w2861 -> [w2880 _]
                  tunnel: w2860 -> [w2879 _]
                  tunnel: w2859 -> [w2878 w3376]
                  frame #0 {
                    # "Effectue la commande ..."
                    n3620 = case shown="\"EOFF\"" w2880 {
                      tunnel: w2879 -> [_ w2886 w2982 w2990 w3029 w3081 w3094 w3110 _ w3295 _]
                      tunnel: w2878 -> [_ _ _ _ _ _ _ _ _ _ _]
                      frame Default {
                        n3621 = local write "ANSW"("Commande non reconnue" ("ANSW")) -> ()
                      }
                      frame "ETCS" {
                        # "Commandes vers TCS"
                        n3622 = call "ETCS_decodeur.vi"("chaine entree"=w2886) -> ("Args"=w2883:dbl[], "nb args"=w2887:i32)  [unwired: 1 out]
                        n3623 = Delete From Array(array=w2883, index=0 ("indice")) -> (deleted portion=w2884:dbl, array with subset deleted=w2882:dbl[])  [unwired: 1 in]
                        n3624 = To Long Integer(number=w2884) -> (32bit integer=w2888:i32)
                        n3625 = case shown="4" w2888 {
                          selector: w2888 -> [_ w2899 _ w2964]
                          tunnel: w2887 -> [_ w2900 w2934 _]
                          tunnel: w2882 -> [_ w2898 _ w2963]
                          frame 0, Default {
                            w2889 = u32 128 ("Bit to add")
                            n3626 = local read "Warning Code"() -> (w2893:u32)
                            n3627 = local read "FIFO d'erreur"() -> (w2891:T7)
                            n3628 = local read "Error Code"() -> (w2892:u32)
                            n3629 = call "Error_Format.vi"("FIFO IN"=w2891, "Error Code IN"=w2892, "Warning Code IN"=w2893, "Error Bit"=w2889, "Warning Bit"=w2889, "Source"="ETCS", "Comment"="Commande non-supportée/indéfinie") -> ("FIFO OUT"=w2894:T7, "Error Code OUT"=w2895:u32, "Warning Code OUT"=w2896:u32)  [unwired: 10 in]
                            n3630 = local write "Warning Code"(w2896) -> ()
                            n3631 = local write "FIFO d'erreur"(w2894) -> ()
                            n3632 = local write "Error Code"(w2895) -> ()
                          }
                          frame 6, 14..16, 22 {
                            # "Vérifie le nombre d'arguments ..."
                            # "Envoir des commandes sans gestions ni réponse de TCS"
                            n3633 = case shown="6" w2899 {
                              tunnel: w2900 -> [w2926 w2927 w2932]
                              tunnel: [w2924 w2928 w2930] -> w2901
                              frame Default {
                                n3634 = Equal?(x=w2926, y=1) -> (x = y?=w2924:bool)
                              }
                              frame 6 {
                                n3635 = Equal?(x=w2927, y=3) -> (x = y?=w2928:bool)
                              }
                              frame 14 {
                                n3636 = Equal?(x=w2932, y=4) -> (x = y?=w2930:bool)
                              }
                            }
                            n3637 = case shown="Vrai" w2901 {
                              tunnel: w2898 -> [_ w2909]
                              tunnel: w2899 -> [_ w2908]
                              frame False {
                                # "Nombre d'arguments incorrect"
                                n3638 = local read "Error Code"() -> (w2904:u32)
                                n3639 = Or(x=w2904, y=u32 128) -> (x .or. y?=w2903:u32)
                                n3640 = local write "Error Code"(w2903) -> ()
                              }
                              frame True {
                                n3641 = local read "TCS VRN"() -> (w2907:refnum<visa-resource-name>)
                                n3642 = control-ref of="TCS actif"() -> (w2905:refnum<vi>)
                                n3643 = call "EXCOM-CMD.vi"("VRN IN"=w2907, "Bool Refnum"=w2905, "Commande #"=w2908, "Args"=w2909) -> ("VRN OUT"=w2906:refnum<visa-resource-name>, "Error OUT"=w2910:errorcluster)  [unwired: 9 in, 1 out]
                                n3644 = local write "TCS VRN"(w2906) -> ()
                                n3645 = case shown="Erreur" w2910 {
                                tunnel: w2908 -> [_ w2921]
                                frame No Error {
                                }
                                frame Error {
                                w2911 = u32 4
                                n3646 = local read "Warning Code"() -> (w2917:u32)
                                n3647 = local read "FIFO d'erreur"() -> (w2919:T7)
                                n3648 = local read "Error Code"() -> (w2918:u32)
                                n3649 = Number To Decimal String(number=w2921) -> (decimal integer string=w2920:string)  [unwired: 1 in]
                                n3650 = Concatenate Strings("Erreur lors de l'envoie de la commande #", w2920, ", vérifiez la communication sur le port TCS C ...") -> (w2916:string)
                                n3651 = call "Error_Format.vi"("FIFO IN"=w2919, "Error Code IN"=w2918, "Warning Code IN"=w2917, "Error Bit"=w2911, "Warning Bit"=w2911, "Source"="ETCS", "Comment"=w2916) -> ("FIFO OUT"=w2915:T7, "Error Code OUT"=w2914:u32, "Warning Code OUT"=w2913:u32)  [unwired: 10 in]
                                n3652 = local write "Warning Code"(w2913) -> ()
                                n3653 = local write "FIFO d'erreur"(w2915) -> ()
                                n3654 = local write "Error Code"(w2914) -> ()
                                }
                                }
                              }
                            }
                          }
                          frame 4 {
                            # "Commande de rotation semie-automatisée ..."
                            n3655 = Equal?(x=w2934, y=2) -> (x = y?=w2935:bool)
                            n3656 = case shown="Vrai" w2935 {
                              frame False {
                                n3657 = local read "Warning Code"() -> (w2942:u32)
                                n3658 = local read "FIFO d'erreur"() -> (w2944:T7)
                                n3659 = local read "Error Code"() -> (w2943:u32)
                                n3660 = call "Error_Format.vi"("FIFO IN"=w2944, "Error Code IN"=w2943, "Warning Code IN"=w2942, "Warning Bit"=u32 128, "Source"="ETCS", "Comment"="Nombre d'arguments incompatibles") -> ("FIFO OUT"=w2940:T7, "Error Code OUT"=w2939:u32, "Warning Code OUT"=w2938:u32)  [unwired: 11 in]
                                n3661 = local write "Warning Code"(w2938) -> ()
                                n3662 = local write "FIFO d'erreur"(w2940) -> ()
                                n3663 = local write "Error Code"(w2939) -> ()
                              }
                              frame True {
                                n3664 = flat-sequence {
                                tunnel: [w2947] -> w2945
                                tunnel: w2945 -> [w2953]
                                frame #0 {
                                w2946 = TRUE ("Value (Signaling)")
                                n3665 = local write "CmdPending"(w2946) -> ()
                                n3666 = property on="ModifRotation" class="Bool (strict)"("Val(Sgnl)"=w2946) -> ()  [unwired: 2 in, 2 out]
                                }
                                frame #1 {
                                n3667 = while {
                                tunnel: [w2948] -> w2947
                                i -> [w2952]
                                stop <- w2951 stop-if-true
                                # "Time-out de 5 minutes ..."
                                n3668 = local read "CmdPending"() -> (w2948:bool)
                                n3669 = Wait (ms)(milliseconds to wait=u32 100) -> ()  [unwired: 1 out]
                                n3670 = call "Max-iteration.vi"("i max"=3000, "i act"=w2952, "Valeur entrante"=w2948) -> ("break ?"=w2951:bool)
                                }
                                }
                                frame #2 {
                                n3671 = case shown="Vrai" w2953 {
                                frame False {
                                }
                                frame True {
                                n3672 = local read "Warning Code"() -> (w2958:u32)
                                n3673 = local read "FIFO d'erreur"() -> (w2960:T7)
                                n3674 = local read "Error Code"() -> (w2959:u32)
                                n3675 = call "Error_Format.vi"("FIFO IN"=w2960, "Error Code IN"=w2959, "Warning Code IN"=w2958, "Warning Bit"=u32 64 ("Bit to add"), "Source"="ETCS", "Comment"="Délai alloué à la commande dépassé !!!") -> ("FIFO OUT"=w2957:T7, "Error Code OUT"=w2956:u32, "Warning Code OUT"=w2955:u32)  [unwired: 11 in]
                                n3676 = local write "Warning Code"(w2955) -> ()
                                n3677 = local write "FIFO d'erreur"(w2957) -> ()
                                n3678 = local write "Error Code"(w2956) -> ()
                                }
                                }
                                }
                                }
                              }
                            }
                          }
                          frame 27 {
                            n3679 = local read "TCS VRN"() -> (w2966:refnum<visa-resource-name>)
                            n3680 = control-ref of="TCS actif"() -> (w2968:refnum<vi>)
                            n3681 = call "EXCOM-CMD.vi"("VRN IN"=w2966, "Bool Refnum"=w2968, "Commande #"=w2964, "Args"=w2963) -> ("VRN OUT"=w2967:refnum<visa-resource-name>, "Error OUT"=w2965:errorcluster)  [unwired: 9 in, 1 out]
                            n3682 = local write "TCS VRN"(w2967) -> ()
                            n3683 = case shown="Erreur" w2965 {
                              tunnel: w2964 -> [_ w2979]
                              frame No Error {
                              }
                              frame Error {
                                w2969 = u32 4
                                n3684 = local read "Warning Code"() -> (w2975:u32)
                                n3685 = local read "FIFO d'erreur"() -> (w2977:T7)
                                n3686 = local read "Error Code"() -> (w2976:u32)
                                n3687 = Number To Decimal String(number=w2979) -> (decimal integer string=w2978:string)  [unwired: 1 in]
                                n3688 = Concatenate Strings("Erreur lors de l'envoie de la commande #", w2978, ", vérifiez la communication sur le port TCS C ...") -> (w2974:string)
                                n3689 = call "Error_Format.vi"("FIFO IN"=w2977, "Error Code IN"=w2976, "Warning Code IN"=w2975, "Error Bit"=w2969, "Warning Bit"=w2969, "Source"="ETCS", "Comment"=w2974) -> ("FIFO OUT"=w2973:T7, "Error Code OUT"=w2972:u32, "Warning Code OUT"=w2971:u32)  [unwired: 10 in]
                                n3690 = local write "Warning Code"(w2971) -> ()
                                n3691 = local write "FIFO d'erreur"(w2973) -> ()
                                n3692 = local write "Error Code"(w2972) -> ()
                              }
                            }
                          }
                        }
                      }
                      frame "ETAB" {
                        n3693 = call "ETAB_decodeur.vi"("chaine entree"=w2982) -> ("Args"=w2983:string[], "OK done"=w2984:bool)  [unwired: 1 out]
                        n3694 = case shown="Vrai" w2984 {
                          tunnel: w2983 -> [_ w2986]
                          frame False {
                          }
